vi "xeva-collect-paramter-error.vi"(2 "error":errorcluster, 3 "xenics-status-cluster-in":T1 caption="xenics-status-cluster") -> (1 "xenics-status-cluster-out":T1 caption="xenics-status-cluster")   [LabVIEW 2015]
panel:
  # "Init"
  # "Cooling"
  # "Parameters"
  # "Xeva"
  # "Init"
  # "Cooling"
  # "Parameters"
  # "Xeva"
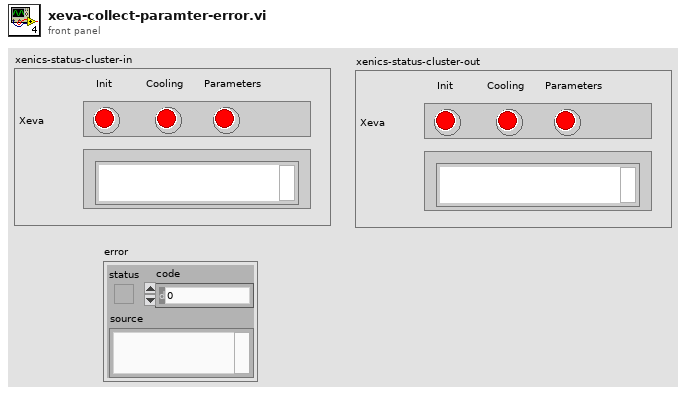
[diagram p1: front panel]
types:
  T1 = cluster{"Xeva-init":bool, "xeva-cooling":bool, "xeva-parameters":bool, "xeva-error":string}
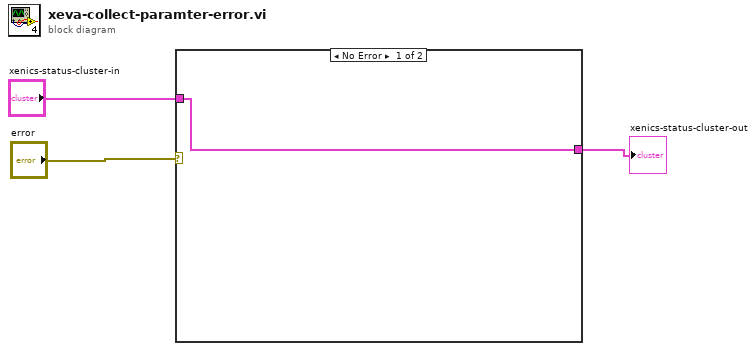
[diagram p0: block diagram]
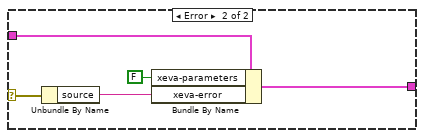
[diagram p2: hidden frame]
diagram:
  n1 = case shown="No Error" "error" {
    selector: "error" -> [_ w8]
    tunnel: "xenics-status-cluster-in" -> [w4 w6]
    tunnel: [w4 w5] -> w1
    frame No Error {
    }
    frame Error {
      n2 = Unbundle By Name(w8) -> ("source"=w7:string)
      n3 = Bundle By Name(cluster=w6, "xeva-parameters"=FALSE, "xeva-error"=w7) -> (w5:T1)
    }
  }
  "xenics-status-cluster-out" <- w1
